vi "Find UUT Record.vi"(8 "error in":errorcluster, 11 "Chronometer in":refnum<class "Chronometer.lvclass">) -> (0 "error out":errorcluster, 3 "Chronometer out":refnum<class "Chronometer.lvclass">)   [LabVIEW 2023, in "Chronometer.lvlib" / "Chronometer.lvclass"]
uses:
  Chronometer.lvclass
  Chronometer.lvclass/Chronometer.ctl
  builds/Tools/Config.lvlibp/Config.lvclass
  C:/Users/Public/Documents/Development/builds/Tools/Config.lvlibp/Config.lvclass
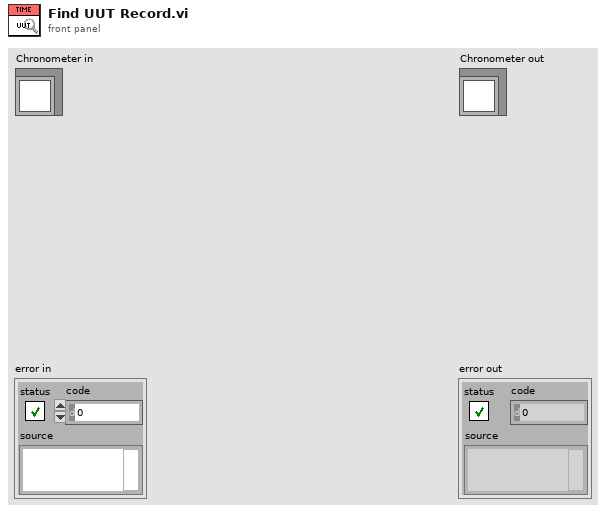
[diagram p1: front panel]
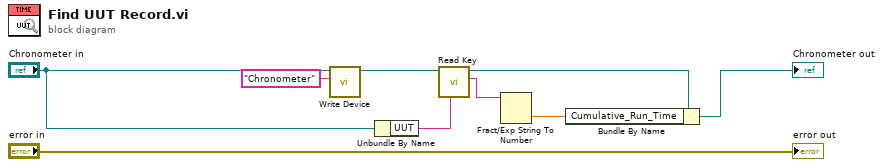
[diagram p0: block diagram]
diagram:
  n1 = call "Write Device.vi"("Device"="Chronometer", "Config in"="Chronometer in") -> ("Config out"=w2:refnum<class "Chronometer.lvclass">)  [unwired: 8 in, 1 out]
  n2 = Unbundle By Name("Chronometer in") -> ("UUT"=w5:string)
  n3 = call "Read Key.vi"("Key Name"=w5, "Config in"=w2) -> ("Key Value"=w4:string, "Config out"=w6:refnum<class "Chronometer.lvclass">)  [unwired: 7 in, 1 out]
  n4 = Fract/Exp String To Number(string=w4) -> (number=w9:dbl)  [unwired: 3 in, 1 out]
  n5 = Bundle By Name(cluster=w6, "Cumulative_Run_Time"=w9) -> (→"Chronometer out":refnum<class "Chronometer.lvclass">)
  "error out" <- "error in"
